vi "Data_Scout_Server.vi"(0 "Relative Path":path) -> (1 "Path":path[](array[path]), 2 "Last Mod":dbl[](array[numeric]), 3 "Size":i64[](array[numeric]))   [LabVIEW 2011]
uses:
  Anemometry/Anemometry Sub Vis/Globals/Constants_global.vi
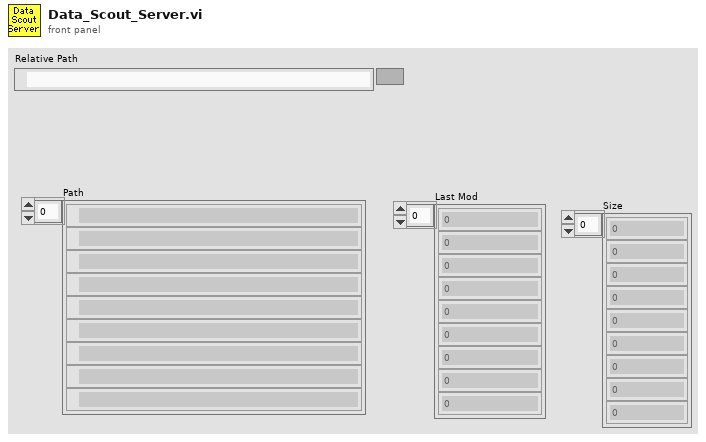
[diagram p1: front panel]
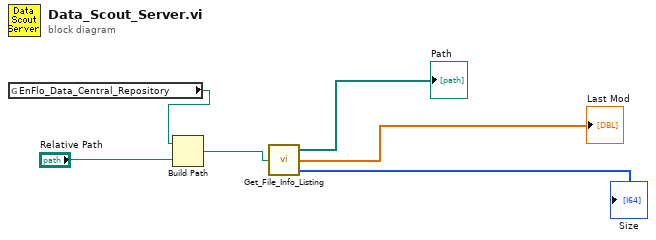
[diagram p0: block diagram]
diagram:
  n1 = global read "Constants_global.vi" "EnFlo_Data_Central_Repository"() -> (w1:path)
  n2 = Build Path(base path=w1, name or relative path="Relative Path") -> (appended path=w2:path)
  n3 = call "Get_File_Info_Listing.vi"("path"=w2) -> ("Path"=→"Path":path[], "Last Mod"=→"Last Mod":dbl[], "Size"=→"Size":i64[])
